vi "stage_dither_region.vi"(6 "first_time":bool, 7 "dither":T1 {"Dither Period (s)" min=0.0; "PVT Ampl (nm)" min=0.0}, 8 "error in (no error)":errorcluster, 9 "cycles":dbl, 10 "Stage Name":string, 11 "newport_xps in":refnum<class "newport_xps.lvclass">) -> (0 "error out":errorcluster, 3 "newport_xps out":refnum<class "newport_xps.lvclass">)   [LabVIEW 2015, in "newport_xps.lvclass"]
uses:
  newport_xps.lvclass
  dither_trajectory_settings.ctl
  dither_trajectory_types.ctl
  newport_xps.lvclass/newport_xps.ctl
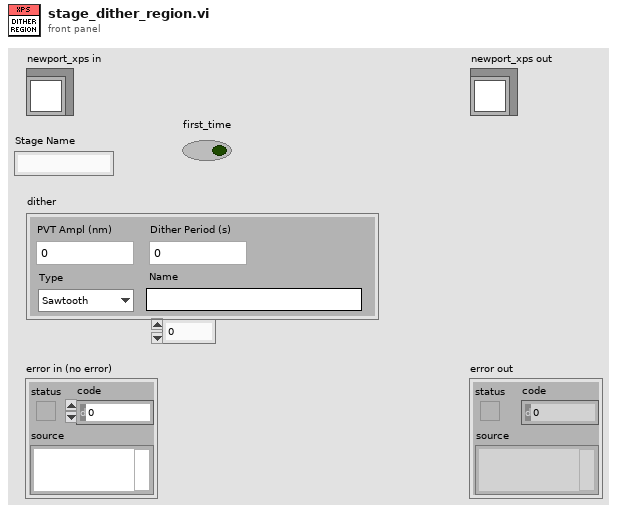
[diagram p1: front panel]
types:
  T1 = typedef "dither_trajectory_settings.ctl" = cluster{"PVT Ampl (nm)":dbl, "Dither Period (s)":dbl, "Type":T2, "Name":string}
  T2 = typedef "dither_trajectory_types.ctl" = enum16{"Sawtooth"}
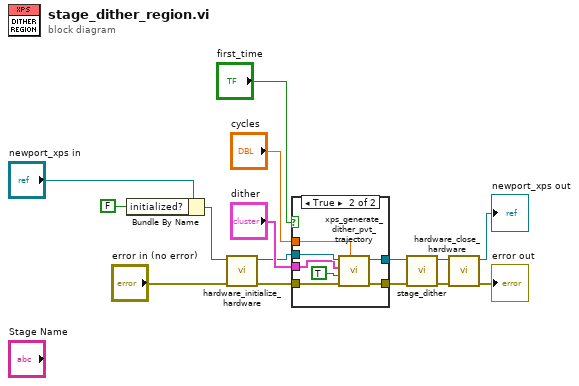
[diagram p0: block diagram]
diagram:
  n1 = Bundle By Name(cluster="newport_xps in", "initialized?"=FALSE) -> (w7:refnum<class "newport_xps.lvclass">)
  n2 = call-dynamic "hardware_initialize_hardware.vi"("error in (no error)"="error in (no error)", "newport_xps in"=w7) -> ("error out"=w1:errorcluster, "newport_xps out"=w6:refnum<class "newport_xps.lvclass">)  [unwired: 8 in]
  n3 = case shown="True" "first_time" {
    tunnel: w1 -> [w16 w24]
    tunnel: w6 -> [w17 w23]
    tunnel: "dither" -> [_ w22]
    tunnel: "cycles" -> [_ w20]
    tunnel: [w17 w19] -> w12
    tunnel: [w16 w18] -> w11
    frame False {
    }
    frame True {
      n4 = call "xps_generate_dither_pvt_trajectory.vi"("Dither Cycles"=w20, "error in (no error)"=w24, "custom?"=TRUE, "Custom Dither Trajectory"=w22, "newport_xps in"=w23) -> ("error out"=w18:errorcluster, "newport_xps out"=w19:refnum<class "newport_xps.lvclass">)  [unwired: 5 in]
    }
  }
  n5 = call-dynamic "stage_dither.vi"("error in (no error)"=w11, "newport_xps in"=w12) -> ("error out"=w2:errorcluster, "newport_xps out"=w5:refnum<class "newport_xps.lvclass">)  [unwired: 8 in]
  n6 = call-dynamic "hardware_close_hardware.vi"("error in (no error)"=w2, "newport_xps in"=w5) -> ("error out"=→"error out":errorcluster, "newport_xps out"=→"newport_xps out":refnum<class "newport_xps.lvclass">)  [unwired: 8 in]
